vi "Main_000.vi"() -> ()   [LabVIEW 2025]
uses:
  Utility/Universal Utility/TypeDefs_Utility/Cluster_Row-Column.ctl
  9e3f57c0-2ef8-4495-8287-c6a42a5fb955.vi
  Utility/Universal Utility/TypeDefs_Utility/ENUM_4 Directions U-D-L-R.ctl
  Utility/Universal Utility/TypeDefs_Utility/ENUM_8 Directions U-D-L-R.ctl
panel:
  out "x-1":u64
  out "Array":u64[](array[numeric])
  out "MATCH":bool
  in  "Select Data":enum32{"Example", "Puzzle"}(tab)
  in  "EX Square Numbers":u64=5
  in  "EX Target":u64=35
  in  "Puzzle Target":u64=66448042666544000
  in  "First Square Numbers":u64=736000
  out "Answer":u64
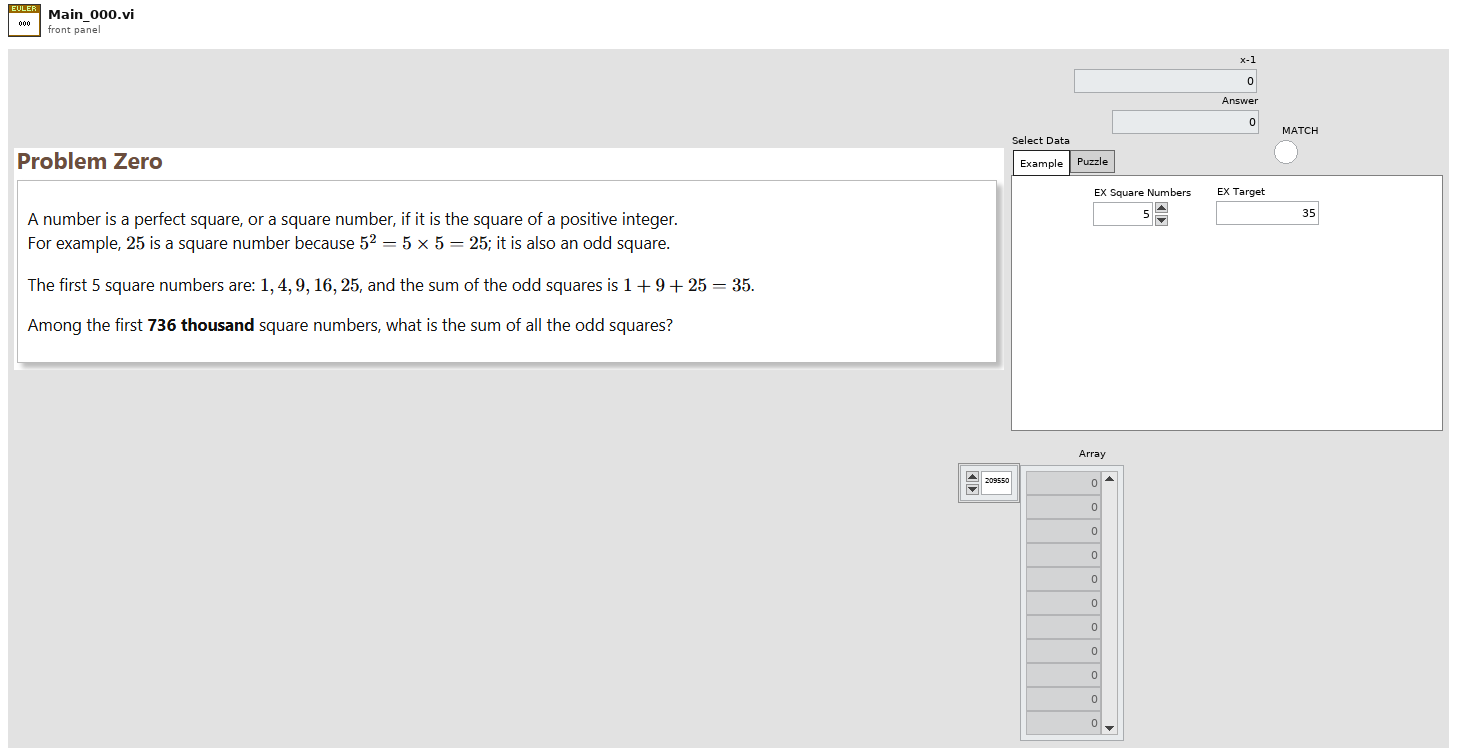
[diagram p1: front panel]
types:
  T1 = typedef "ENUM_8 Directions U-D-L-R.ctl" = enum16{"Up;-1,0", "Up-Right;-1,1", "Right;0,1", "Down-Right;1,1", "Down;1,0", "Down-Left;1,-1", "Left;0,-1", "Up-Left;-1,-1"}
  T2 = typedef "ENUM_4 Directions U-D-L-R.ctl" = enum16{"Up;-1,0", "Right;0,1", "Down;1,0", "Left;0,-1"}
  T3 = typedef "Cluster_Row-Column.ctl" = cluster{"R":i32, "C":i32}
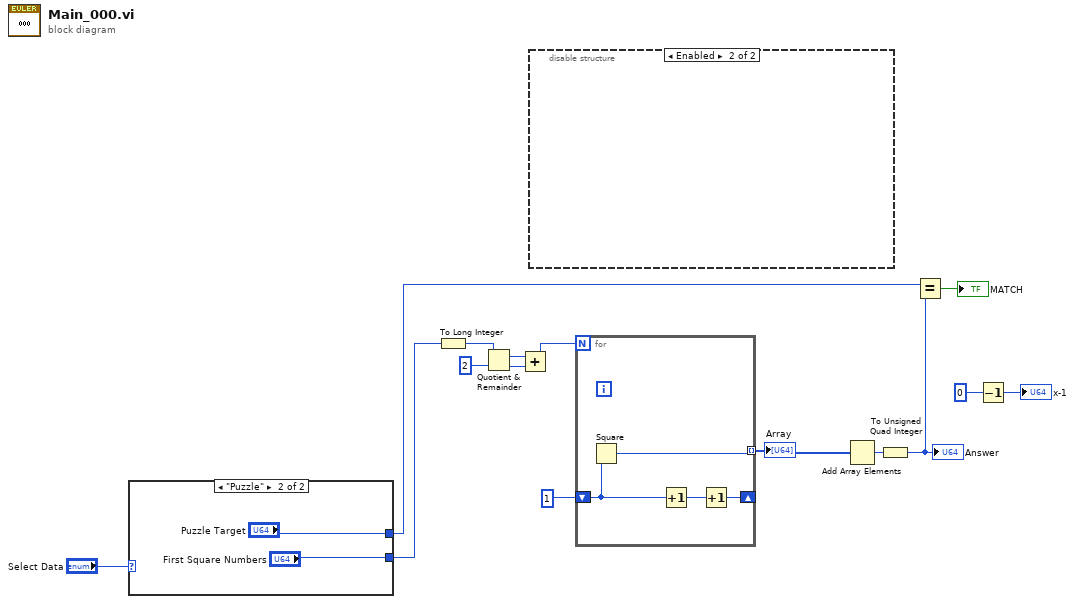
[diagram p0: block diagram]
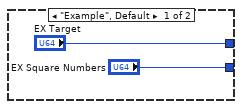
[diagram p2: hidden frame]
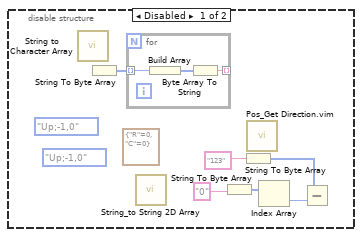
[diagram p3: hidden frame]
diagram:
  n1 = case shown="\"Puzzle\"" "Select Data" {
    tunnel: ["EX Square Numbers" "First Square Numbers"] -> w11
    tunnel: ["EX Target" "Puzzle Target"] -> w13
    frame "Example", Default {
    }
    frame "Puzzle" {
    }
  }
  n2 = To Long Integer(number=w11) -> (32bit integer=w7:i32)
  n3 = Quotient & Remainder(x=w7, y=2) -> (x-y*floor(x/y)=w9:i32, floor(x/y)=w8:i32)
  n4 = Add(x=w9, y=w8) -> (x+y=w6:i32)
  n5 = disable-structure shown="Enabled" {
    frame Disabled {
      (unwired) ENUM_8_Directions_U-D-L-R."Up;-1,0" ("Direction 8")
      (unwired) ENUM_4_Directions_U-D-L-R."Up;-1,0" ("Direction")
      (unwired) T3 {"R"=0, "C"=0} ("Position")
      n6 = call "String to Character Array.vi"() -> ()  [unwired: 1 in, 1 out]
      n7 = String To Byte Array() -> (unsigned byte array=w20:u8[])  [unwired: 1 in]
      n8 = for {
        tunnel: w20 -> [w28] mode=indexing
        tunnel: [w26] -> _ mode=indexing
        n9 = Build Array(w28) -> (w27:u8[])
        n10 = Byte Array To String(unsigned byte array=w27) -> (string=w26:string)
      }
      n11 = call "String_to String 2D Array.vi"() -> ()  [unwired: 11 in, 1 out]
      n12 = String To Byte Array(string="0") -> (unsigned byte array=w23:u8[])
      n13 = String To Byte Array(string="123") -> (unsigned byte array=w21:u8[])
      n14 = call "Pos_Get Direction.vim"() -> ()  [unwired: 11 in, 1 out]
      n15 = Index Array(array=w23) -> (element=w22:u8)  [unwired: 1 in]
      n16 = Subtract(x=w21, y=w22) -> ()  [unwired: 1 out]
    }
    frame Enabled {
    }
  }
  n17 = for {
    N: w6 -> [_]
    shift-right: [w31] -> _
    shift-left: u64 1 ("y") -> [w30]
    tunnel: [w29] -> w4 mode=indexing
    n18 = Square(x=w30) -> (x^2=w29:u64)
    n19 = Increment(x=w30) -> (x+1=w32:u64)
    n20 = Increment(x=w32) -> (x+1=w31:u64)
  }
  "Array" <- w4
  n21 = Add Array Elements(numeric array=w4) -> (sum=w3:u64)
  n22 = To Unsigned Quad Integer(1:w3) -> (0:w12:u64)
  "Answer" <- w12
  n23 = Equal?(x=w13, y=w12) -> (x = y?=→"MATCH":bool)
  n24 = Decrement(x=u64 0 ("unsigned 64bit integer")) -> (x-1=→"x-1":u64)
